vi "ReadLogRolloverNode.vi"(8 "Error In":errorcluster, 11 "Keithley2602 Node In":refnum<k20>) -> (0 "Error Out":errorcluster, 2 "Log Rollover Configuration":T1, 3 "Keithley2602 Node Out":refnum<k20>)   [LabVIEW 2012]
uses:
  LogRolloverConfiguration.ctl
  LogRolloverTriggerType.ctl
  LogDigitalIOTriggerEdge.ctl
  <vilib>/xml/NI_XML.lvlib
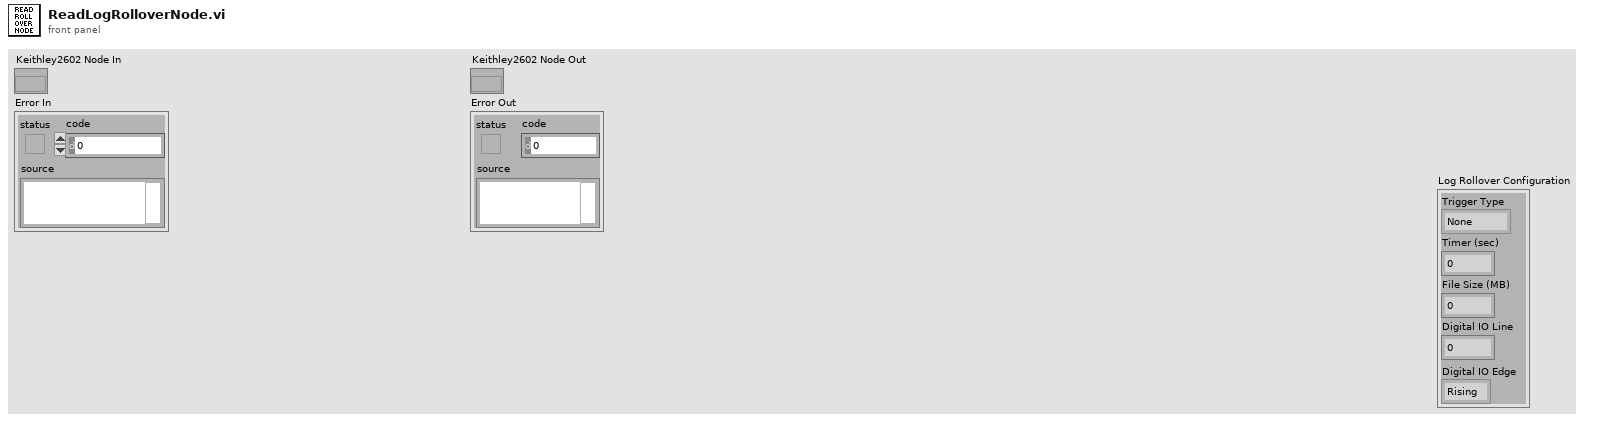
[diagram p1: front panel]
types:
  T1 = typedef "LogRolloverConfiguration.ctl" = cluster{"Trigger Type":T2, "Timer (sec)":dbl, "File Size (MB)":u32, "Digital IO Line":u8, "Digital IO Edge":T3}
  T2 = typedef "LogRolloverTriggerType.ctl" = enum16{"None", "Timer", "File Size", "Digital IO"}
  T3 = typedef "LogDigitalIOTriggerEdge.ctl" = enum16{"Rising", "Falling"}
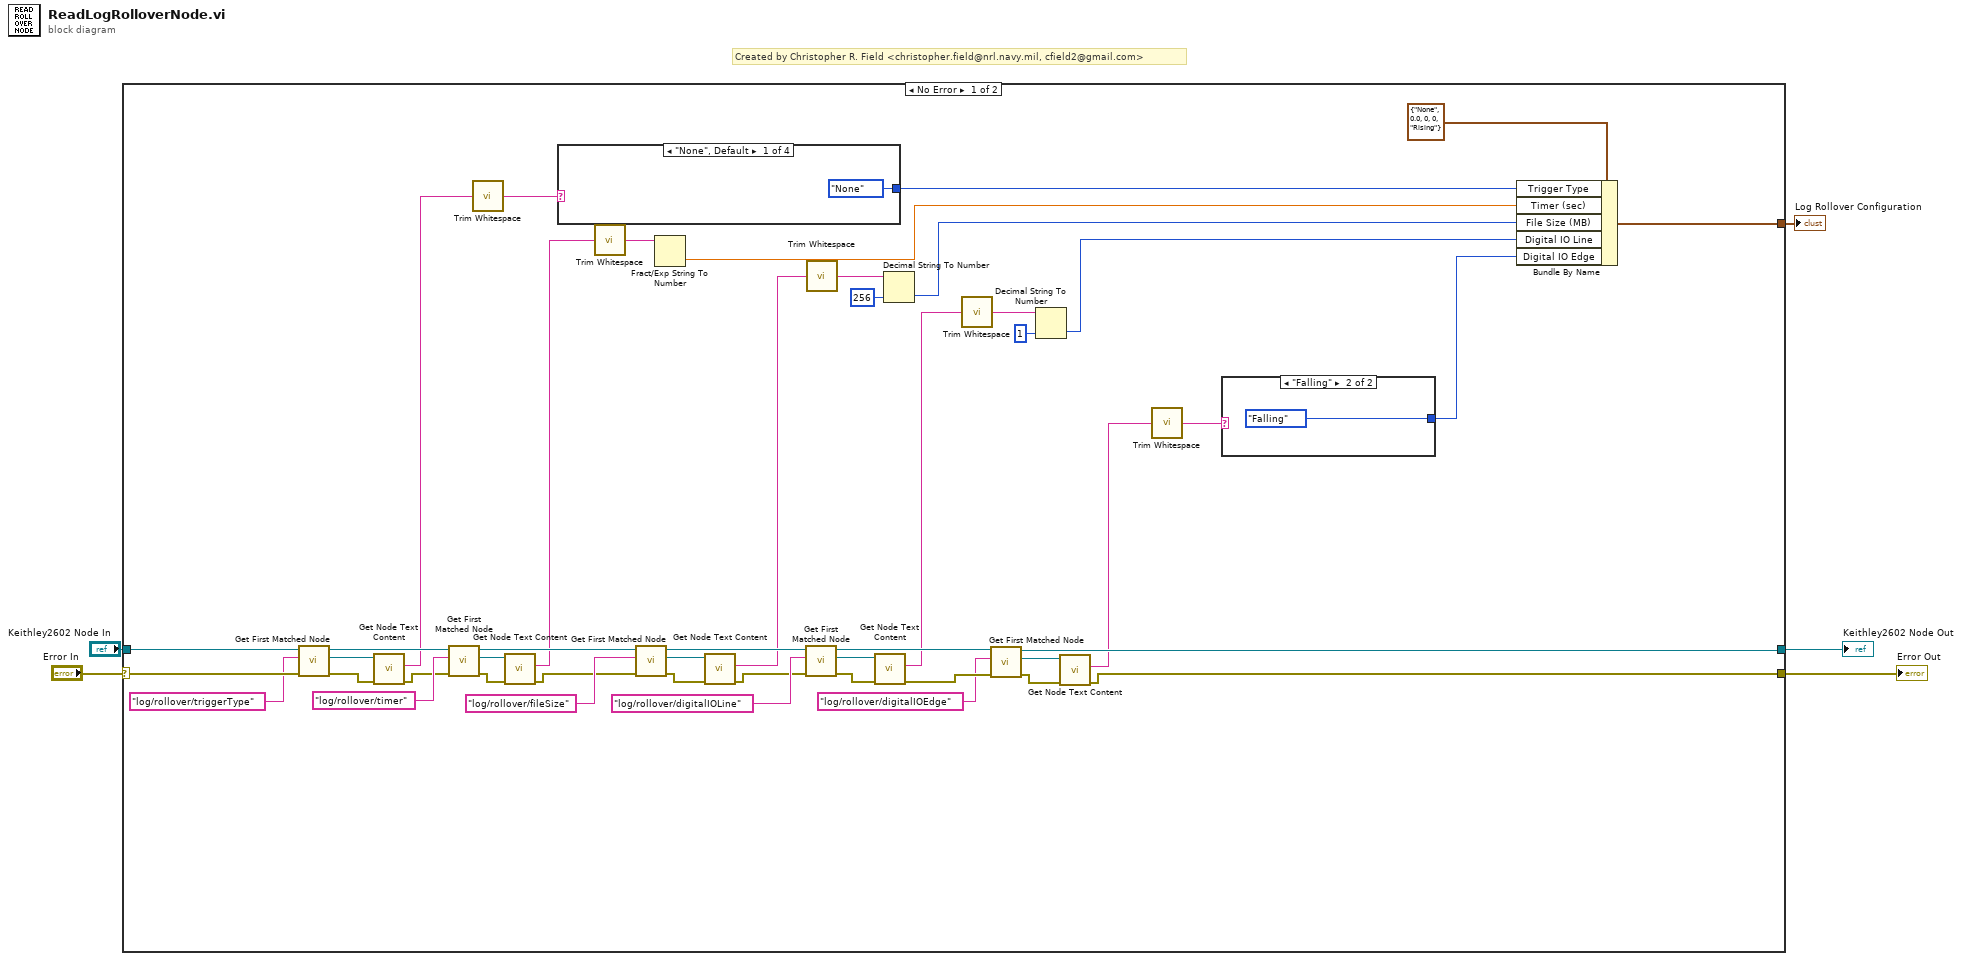
[diagram p0: block diagram]
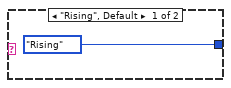
[diagram p2: hidden frame]
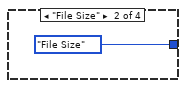
[diagram p3: hidden frame]
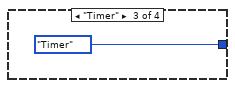
[diagram p4: hidden frame]
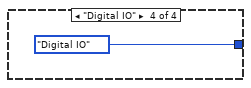
[diagram p5: hidden frame]
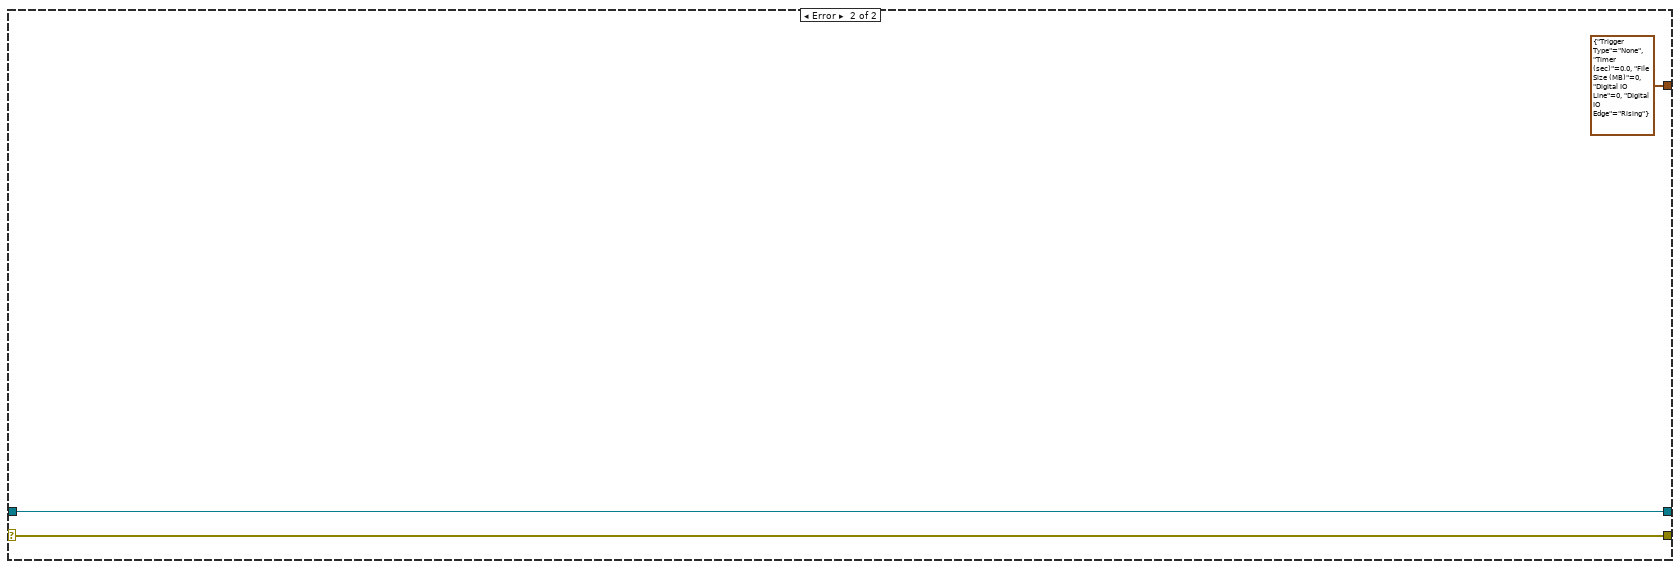
[diagram p6: hidden frame]
diagram:
  # "Created by Christopher R. Field <christopher.field@nrl.navy.mil, cfield2@gmail.com>"
  n1 = case shown="No Error" "Error In" {
    selector: "Error In" -> [w50 w59]
    tunnel: "Keithley2602 Node In" -> [w51 w60]
    tunnel: [w32 w60] -> w3
    tunnel: [w31 w59] -> w2
    tunnel: [w29 T1 {"Trigger Type"=enum."None", "Timer (sec)"=0.0, "File Size (MB)"=0, "Digital IO Line"=0, "Digital IO Edge"=enum."Rising"} ("Log Rollover Configuration")] -> w1
    frame No Error {
      n2 = call <vilib>:"Get First Matched Node.vi"("error in (no error)"=w50, "XPath expression"="log/rollover/triggerType", "node in"=w51) -> ("error out"=w47:errorcluster, "node result"=w48:refnum<k20>, "node out"=w45:refnum<k20>)  [unwired: 6 in]
      n3 = call <vilib>:"Get Node Text Content.vi"("error in (no error)"=w47, "node in"=w48) -> ("error out"=w44:errorcluster, "node text"=w14:string)  [unwired: 7 in, 1 out]
      n4 = call <vilib>:"Get First Matched Node.vi"("error in (no error)"=w44, "XPath expression"="log/rollover/timer", "node in"=w45) -> ("error out"=w42:errorcluster, "node result"=w43:refnum<k20>, "node out"=w27:refnum<k20>)  [unwired: 6 in]
      n5 = call <vilib>:"Trim Whitespace.vi"("string"=w14) -> ("trimmed string"=w15:string)  [unwired: 1 in]
      n6 = call <vilib>:"Get Node Text Content.vi"("error in (no error)"=w42, "node in"=w43) -> ("error out"=w21:errorcluster, "node text"=w12:string)  [unwired: 7 in, 1 out]
      n7 = case shown="\"None\", Default" w15 {
        tunnel: [LogRolloverTriggerType."None" ("Trigger Type") LogRolloverTriggerType."File Size" ("Trigger Type") LogRolloverTriggerType."Timer" ("Trigger Type") LogRolloverTriggerType."Digital IO" ("Trigger Type")] -> w28
        frame "None", Default {
        }
        frame "File Size" {
        }
        frame "Timer" {
        }
        frame "Digital IO" {
        }
      }
      n8 = call <vilib>:"Trim Whitespace.vi"("string"=w12) -> ("trimmed string"=w13:string)  [unwired: 1 in]
      n9 = call <vilib>:"Get First Matched Node.vi"("error in (no error)"=w21, "XPath expression"="log/rollover/fileSize", "node in"=w27) -> ("error out"=w25:errorcluster, "node result"=w26:refnum<k20>, "node out"=w23:refnum<k20>)  [unwired: 6 in]
      n10 = Fract/Exp String To Number(string=w13) -> (number=w20:dbl)  [unwired: 3 in, 1 out]
      n11 = call <vilib>:"Get Node Text Content.vi"("error in (no error)"=w25, "node in"=w26) -> ("error out"=w22:errorcluster, "node text"=w10:string)  [unwired: 7 in, 1 out]
      n12 = call <vilib>:"Get First Matched Node.vi"("error in (no error)"=w22, "XPath expression"="log/rollover/digitalIOLine", "node in"=w23) -> ("error out"=w39:errorcluster, "node result"=w40:refnum<k20>, "node out"=w35:refnum<k20>)  [unwired: 6 in]
      n13 = call <vilib>:"Trim Whitespace.vi"("string"=w10) -> ("trimmed string"=w11:string)  [unwired: 1 in]
      n14 = call <vilib>:"Get Node Text Content.vi"("error in (no error)"=w39, "node in"=w40) -> ("error out"=w34:errorcluster, "node text"=w8:string)  [unwired: 7 in, 1 out]
      n15 = Decimal String To Number(string=w11, default (0L)=u32 256 ("default (0 I32)")) -> (number=w18:u32)  [unwired: 1 in, 1 out]
      n16 = call <vilib>:"Trim Whitespace.vi"("string"=w8) -> ("trimmed string"=w9:string)  [unwired: 1 in]
      n17 = call <vilib>:"Get First Matched Node.vi"("error in (no error)"=w34, "XPath expression"="log/rollover/digitalIOEdge", "node in"=w35) -> ("error out"=w36:errorcluster, "node result"=w37:refnum<k20>, "node out"=w32:refnum<k20>)  [unwired: 6 in]
      n18 = Decimal String To Number(string=w9, default (0L)=u32 1 ("default (0 I32)")) -> (number=w17:u32)  [unwired: 1 in, 1 out]
      n19 = call <vilib>:"Get Node Text Content.vi"("error in (no error)"=w36, "node in"=w37) -> ("error out"=w31:errorcluster, "node text"=w6:string)  [unwired: 7 in, 1 out]
      n20 = call <vilib>:"Trim Whitespace.vi"("string"=w6) -> ("trimmed string"=w7:string)  [unwired: 1 in]
      n21 = case shown="\"Falling\"" w7 {
        tunnel: [LogDigitalIOTriggerEdge."Rising" ("Digital IO Edge") LogDigitalIOTriggerEdge."Falling" ("Digital IO Edge")] -> w16
        frame "Rising", Default {
        }
        frame "Falling" {
        }
      }
      n22 = Bundle By Name(cluster=T1 {"Trigger Type"=enum."None", "Timer (sec)"=0.0, "File Size (MB)"=0, "Digital IO Line"=0, "Digital IO Edge"=enum."Rising"} ("Log Rollover Configuration"), "Trigger Type"=w28, "Timer (sec)"=w20, "File Size (MB)"=w18, "Digital IO Line"=w17, "Digital IO Edge"=w16) -> (w29:T1)
    }
    frame Error {
    }
  }
  "Keithley2602 Node Out" <- w3
  "Error Out" <- w2
  "Log Rollover Configuration" <- w1
